vi "Exchange for Access Token.vi"(8 "error in (no error)":errorcluster, 9 "OAuth Credentials (request)":T1={"Signature Method"=enum."HMAC-SHA1", "Version"="", "Client"={"Token"="", "Secret"=""}, "Access"={"Token"="", "Secret"=""}}, 10 "Pin":string, 11 "Access Request URL":string) -> (0 "error out":errorcluster, 1 "OAuth Credentials (access)":T1={"Signature Method"=enum."HMAC-SHA1", "Version"="", "Client"={"Token"="", "Secret"=""}, "Access"={"Token"="", "Secret"=""}}, 2 "body":string, 3 "headers":string)   [LabVIEW 2011, in "i3-oauth.lvlib"]
doc: "Uses a PIN to exchange an OAuth request token and token secret for an OAuth access token and token secret."
uses:
  i3-oauth.lvlib
  Controls/OAuth Handle.ctl
  Controls/Signature Method.ctl
  Controls/Credentials.ctl
  Controls/HTTP Method.ctl
  <vilib>/httpClient/POSTBuffer.vi
  <vilib>/httpClient/LabVIEWHTTPClient.lvlib
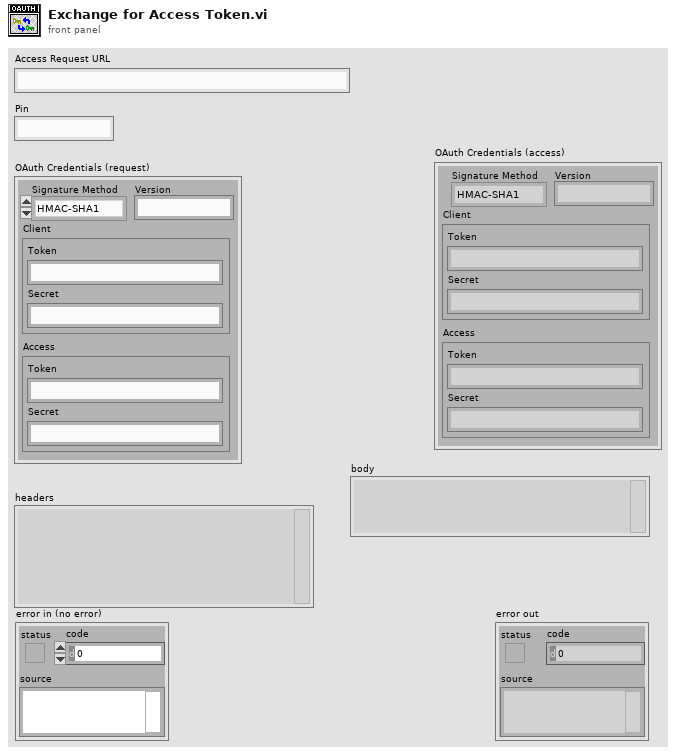
[diagram p1: front panel]
types:
  T1 = typedef "i3-oauth.lvlib/OAuth Handle.ctl" = cluster{"Signature Method":T2, "Version":string, "Client":T3, "Access":T3}
  T2 = typedef "i3-oauth.lvlib/Signature Method.ctl" = enum16{"HMAC-MD5", "HMAC-SHA1", "HMAC-SHA224", "HMAC-SHA256", "HMAC-SHA384", "HMAC-SHA512"}
  T3 = typedef "i3-oauth.lvlib/Credentials.ctl" = cluster{"Token":string, "Secret":string}
  T4 = typedef "i3-oauth.lvlib/HTTP Method.ctl" = enum16{"GET", "POST", "PUT", "DELETE"}
  T5 = typedef "i3-oauth.lvlib/Name-Value Pair.ctl" = cluster{"Name":string, "Value":string}
  T6 = typedef "LabVIEWHTTPClient.lvlib/ClientHandle.ctl" = refnum<k1>
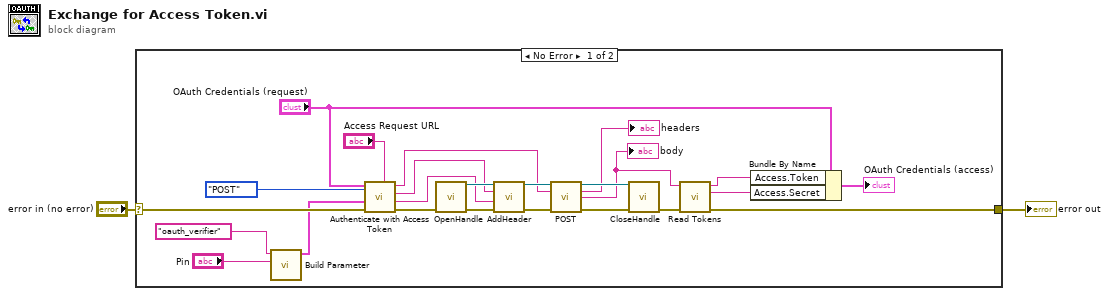
[diagram p0: block diagram]
diagram:
  n1 = case shown="No Error" "error in (no error)" {
    selector: "error in (no error)" -> [w25 w26]
    tunnel: [w6 w26] -> w1
    frame No Error {
      n2 = call "Build Parameter.vi"("Value"="Pin", "Key"="oauth_verifier" ("key")) -> ("Parameter Array"=w7:T5[])  [unwired: 9 in]
      n3 = call "Authenticate with Access Token.vi"("Base URL"="Access Request URL", "HTTP Method"=HTTP_Method."POST", "error in (no error)"=w25, "Header Parameters"=w7, "OAuth Handle"="OAuth Credentials (request)") -> ("error out"=w10:errorcluster, "Header Value"=w11:string, "Header Parameter"=w12:string, "Full URL"=w8:string)  [unwired: 2 in, 1 out]
      n4 = call <vilib>:"OpenHandle.vi"() -> ("client handle out"=w13:T6)  [unwired: 14 in, 1 out]
      n5 = call <vilib>:"AddHeader.vi"("client handle"=w13, "header"=w12, "value"=w11, "error in (no error)"=w10) -> ("client handle out"=w14:T6, "error out"=w9:errorcluster)  [unwired: 10 in]
      n6 = call-poly <vilib>:"POST.vi"("client handle"=w14, "url"=w8, "error in (no error)"=w9) -> ("client handle out"=w23:T6, "headers"=→"headers":string, "body"=w17:string, "error out"=w24:errorcluster)  [unwired: 9 in]
      "body" <- w17
      n7 = call <vilib>:"CloseHandle.vi"("client handle"=w23, "error in (no error)"=w24) -> ("error out"=w20:errorcluster)  [unwired: 13 in]
      n8 = call "Read Tokens.vi"("error in (no error)"=w20, "input string"=w17) -> ("error out"=w6:errorcluster, "Token Secret"=w18:string, "Token"=w19:string)  [unwired: 7 in]
      n9 = Bundle By Name(cluster="OAuth Credentials (request)", "Access.Token"=w19, "Access.Secret"=w18) -> (→"OAuth Credentials (access)":T1)
    }
    frame Error {
    }
  }
  "error out" <- w1
